vi "Power Accuracy Close Test.vi"(6 "Driver Refs":T3, 8 "error in (no error)":errorcluster) -> (0 "error out":errorcluster {"code" format="%.0x"})   [LabVIEW 2011]
uses:
  drivers/PIM/PIM Driver Ref.ctl
  drivers/PWM/PWM Driver Ref.ctl
  drivers/PIM/PIM Command.ctl
  drivers/PWM/PWM Command.ctl
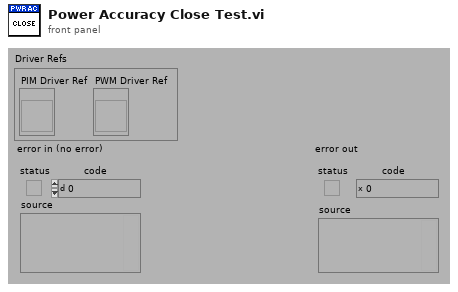
[diagram p1: front panel]
types:
  T1 = typedef "PIM Driver Ref.ctl" = refnum<vi>
  T2 = typedef "PWM Driver Ref.ctl" = refnum<vi>
  T3 = cluster{"PIM Driver Ref":T1, "PWM Driver Ref":T2}
  T4 = typedef "PWM Command.ctl" = enum16{"LOAD", "INITIALIZE", "PRESET", "GET STIMULUS", "SET STIMULUS", "MEASURE", "RELEASE", "UNLOAD", "GET CALIBRATION", "CALIBRATE"}
  T5 = typedef "PIM Command.ctl" = enum16{"LOAD", "KEEP ALIVE", "VALIDATE", "INITIALIZE", "PRESET", "GET CALIBRATION", "SET STIMULUS", "TOGGLE TX POWER", "SET TX ON", "SET TX OFF", "MEASURE", "UNLOAD"}
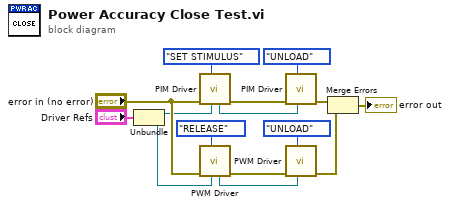
[diagram p0: block diagram]
diagram:
  n1 = Unbundle("Driver Refs") -> ("PIM Driver Ref"=w1:T1, "PWM Driver Ref"=w3:T2)
  n2 = call "PIM Driver.vi"("Driver Ref (null)"=w1, "PIM Command"=PIM_Command."SET STIMULUS" ("DMM Command"), "error in (no error)"="error in (no error)") -> ("error out"=w10:errorcluster, "duplicate driver ref"=w8:T1)  [unwired: 5 in, 2 out]
  n3 = call "PWM Driver.vi"("Drv Refnum"=w3, "PWM Command"=PWM_Command."RELEASE", "error in (no error)"="error in (no error)") -> ("error out"=w11:errorcluster, "dup Drv Refnum"=w7:T2)  [unwired: 5 in, 2 out]
  n4 = call "PIM Driver.vi"("Driver Ref (null)"=w8, "PIM Command"=PIM_Command."UNLOAD" ("DMM Command"), "error in (no error)"=w10) -> ("error out"=w6:errorcluster)  [unwired: 5 in, 3 out]
  n5 = call "PWM Driver.vi"("Drv Refnum"=w7, "PWM Command"=PWM_Command."UNLOAD", "error in (no error)"=w11) -> ("error out"=w5:errorcluster)  [unwired: 5 in, 3 out]
  n6 = Merge Errors(w6, w5) -> (→"error out":errorcluster)
